vi "Copy Array to Image (ARGB).vi"(7 "Set Alpha Values to 255 (Default: True)":bool=TRUE, 8 "error in (no error)":errorcluster, 10 "ARGB Image Destination in":T1, 11 "U32 ARBG Data":u32[][](array[numeric])) -> (0 "error out":errorcluster, 3 "ARGB Image Destination":T1)   [LabVIEW 2020, in "image.lvlib"]
doc: "Copy 2D ARGB Data into the Destination Image. The Destination Image will be resized to fit the Array Data."
uses:
  image.lvlib
  ARGB Image.ctl
  common/common.lvlib
  common/bin/gartoolkit_32-1.dll
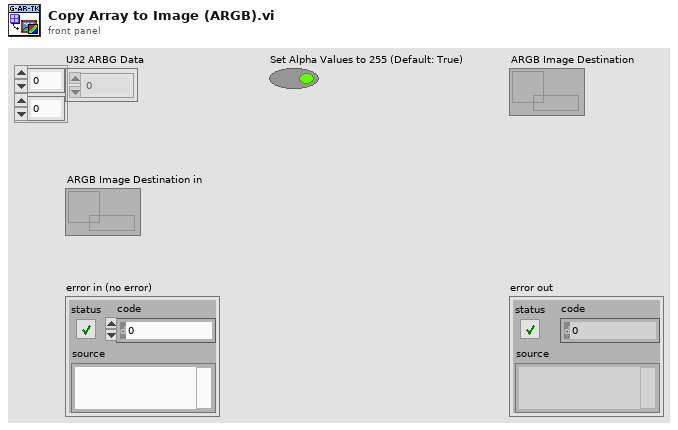
[diagram p1: front panel]
types:
  T1 = typedef "image.lvlib/ARGB Image.ctl" = refnum<data-value>
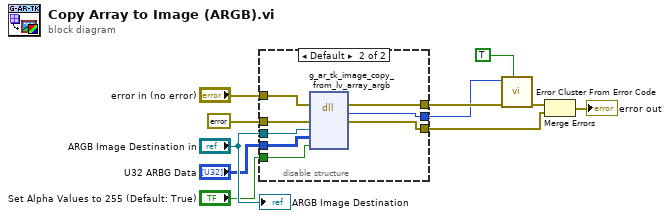
[diagram p0: block diagram]
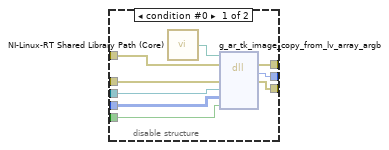
[diagram p2: hidden frame]
diagram:
  n1 = disable-structure shown="Default" {
    disable-tunnel: "error in (no error)" -> [w20 w28]
    disable-tunnel: errorcluster {"status"=FALSE, "code"=0, "source"=""} ("error constant") -> [w19 w27]
    disable-tunnel: "ARGB Image Destination in" -> [w18 w26]
    disable-tunnel: "U32 ARBG Data" -> [w17 w25]
    disable-tunnel: "Set Alpha Values to 255 (Default: True)" -> [w16 w24]
    disable-tunnel: [w15 w23] -> w4
    disable-tunnel: [w14 w22] -> w3
    disable-tunnel: [w13 w21] -> w2
    frame condition #0 {
      n2 = call "NI-Linux-RT Shared Library Path (Core).vi"() -> ("Path"=w12:path)
      n3 = dll-call lib="?" fn="g_ar_tk_image_copy_from_lv_array_argb" ("g_ar_toolkit.*.*:g_ar_tk_image_copy_from_raw_memory")(path in=w12, error in=w20, "error_cluster"=w19, "edvr_dst"=w18, "array"=w17, "set_alpha_255"=w16) -> (error out=w15:errorcluster, w14:i32, "error_cluster"=w13:errorcluster)  [unwired: 4 in, 1 out]
    }
    frame condition #1 (active) {
      n4 = dll-call lib="C:/serenial/lib/g-augmented-reality-toolkit/LabVIEW/common/bin/gartoolkit_*-1.*" fn="g_ar_tk_image_copy_from_lv_array_argb" ("g_ar_toolkit.*.*:g_ar_tk_image_copy_from_raw_memory")(error in=w28, "error_cluster"=w27, "edvr_dst"=w26, "array"=w25, "set_alpha_255"=w24) -> (error out=w23:errorcluster, w22:i32, "error_cluster"=w21:errorcluster)  [unwired: 5 in, 1 out]
    }
  }
  n5 = call <vilib>:"Error Cluster From Error Code.vi"("show call chain? (False)"=TRUE, "error in (no error)"=w4, "error code (0)"=w3) -> ("error out"=w10:errorcluster)  [unwired: 6 in]
  n6 = Merge Errors(w10, w2) -> (→"error out":errorcluster)
  "ARGB Image Destination" <- "ARGB Image Destination in"
